vi "Configure Transform Window.vi"(6 "Step Rise Time (1E-10 s)":dbl=1e-10, 7 "Impulse Width (1E-9 s)":dbl=1e-09, 8 "error in (no error)":errorcluster, 9 "Kaiser Bessel Width (6)":dbl=6.0, 10 "Channel (1)":i32=1, 11 "VISA resource name":refnum<visa-resource-name>) -> (0 "error out":errorcluster, 3 "VISA resource name out":refnum<visa-resource-name>)   [LabVIEW 2018, in "Keysight PNA Series.lvlib"]
doc: "Configures the transform window."
uses:
  Keysight PNA Series.lvlib
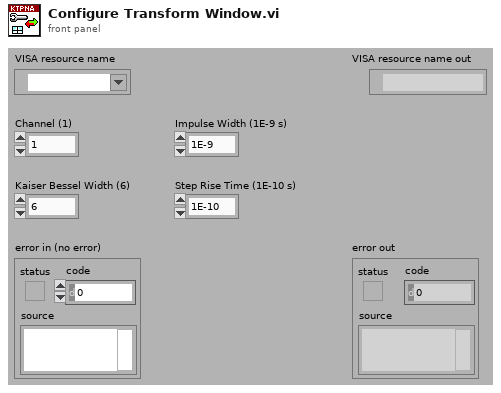
[diagram p1: front panel]
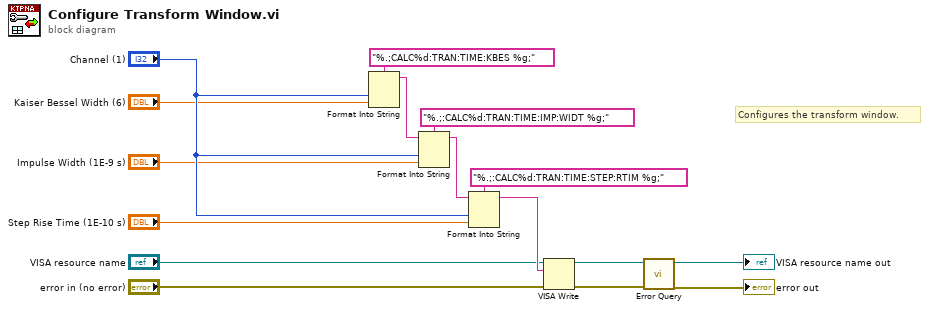
[diagram p0: block diagram]
diagram:
  # "Configures the transform window."
  n1 = Format Into String(format string="%.;CALC%d:TRAN:TIME:KBES %g;", "Channel (1)", "Kaiser Bessel Width (6)") -> (resulting string=w13:string)  [unwired: 2 in, 1 out]
  n2 = Format Into String(format string="%.;:CALC%d:TRAN:TIME:IMP:WIDT %g;", initial string=w13, "Channel (1)", "Impulse Width (1E-9 s)") -> (resulting string=w10:string)  [unwired: 1 in, 1 out]
  n3 = Format Into String(format string="%.;:CALC%d:TRAN:TIME:STEP:RTIM %g;", initial string=w10, "Channel (1)", "Step Rise Time (1E-10 s)") -> (resulting string=w7:string)  [unwired: 1 in, 1 out]
  n4 = VISA Write(VISA resource name="VISA resource name", write buffer=w7, error in (no error)="error in (no error)") -> (VISA resource name out=w4:refnum<visa-resource-name>, error out=w3:errorcluster)  [unwired: 1 out]
  n5 = call "Error Query.vi"("error in (no error)"=w3, "VISA resource name"=w4) -> ("error out"=→"error out":errorcluster, "VISA resource name out"=→"VISA resource name out":refnum<visa-resource-name>)  [unwired: 6 in, 2 out]
